vi "Launch TCP Server and Client Sample Project.vi"   [LabVIEW 2017]
uses:
  Workers/TCP Client Example/Initialization Data.ctl
  Workers/TCP Client Example/TCP Client Example.lvclass
panel:
  # "Running this VI will load three Workers applications asynchronously.\nIt will load:\n\nOne instance of the TCP Server Example application\nTwo instances of the TCP Client Example application\n\nBefore running this VI, look at the code and comments on this VI's block diagram"
types:
  T1 = typedef "TCP Client Example.lvclass/Initialization Data.ctl" = cluster{"Client Name":string}
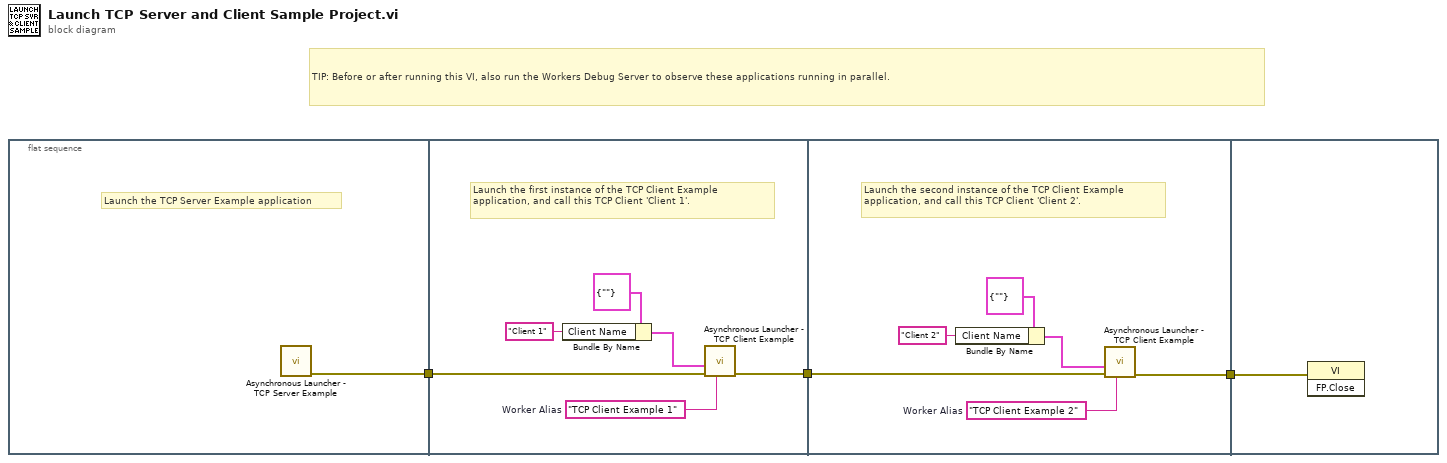
[diagram p0: block diagram]
diagram:
  # "TIP: Before or after running this VI, also run the Workers Debug Server to observe these applications running in parallel."
  n1 = flat-sequence {
    tunnel: [w4] -> w3
    tunnel: w3 -> [w6]
    tunnel: [w5] -> w2
    tunnel: w2 -> [w12]
    tunnel: [w11] -> w1
    tunnel: w1 -> [w17]
    frame #0 {
      # "Launch the TCP Server Example application"
      n2 = call "Asynchronous Launcher - TCP Server Example.vi"() -> ("error out"=w4:errorcluster)  [unwired: 10 in, 1 out]
    }
    frame #1 {
      w7 = "TCP Client Example 1"  # Worker Alias
      # "Launch the first instance of the TCP Client Example application, and call this TCP Client 'Client 1'."
      n3 = Bundle By Name(cluster=T1 {"Client Name"=""} ("Initialization Data"), "Client Name"="Client 1") -> (w10:T1)
      n4 = call "Asynchronous Launcher - TCP Client Example.vi"("Worker Alias"=w7, "error in"=w6, "Initialization Data"=w10) -> ("error out"=w5:errorcluster)  [unwired: 7 in, 1 out]
    }
    frame #2 {
      w13 = "TCP Client Example 2"  # Worker Alias
      # "Launch the second instance of the TCP Client Example application, and call this TCP Client 'Client 2'."
      n5 = Bundle By Name(cluster=T1 {"Client Name"=""} ("Initialization Data"), "Client Name"="Client 2") -> (w16:T1)
      n6 = call "Asynchronous Launcher - TCP Client Example.vi"("Worker Alias"=w13, "error in"=w12, "Initialization Data"=w16) -> ("error out"=w11:errorcluster)  [unwired: 7 in, 1 out]
    }
    frame #3 {
      n7 = invoke class="VI" method="FP.Close"(error in=w17) -> ()  [unwired: 2 in, 3 out]
    }
  }
